vi "Send Publisher Instance Return.vi"(8 "error in (no error)":errorcluster, 10 "Publisher Instance":T1, 11 "CIFChannelMng in":refnum<class "CIFChannelMng.lvclass">) -> (0 "error out":errorcluster, 3 "CIFChannelMng out":refnum<class "CIFChannelMng.lvclass">)   [LabVIEW 2021, in "CIFChannelMng.lvclass"]
uses:
  CIFChannelMng.lvclass
  OOB/OOB_Tx/Typedef/FIFO Publisher Return.ctl
  CIFChannelMng.lvclass/CIFChannelMng.ctl
  <vilib>/CIF Foundation/CIF Out of Band Commands/CIFOutOfBand.lvclass/CIFOutOfBand.ctl
  <vilib>/CIF Foundation/CIF Out of Band Commands/Queue Command.vi
  <vilib>/CIF Foundation/CIF Out of Band Commands/Utilities/Command to Bitwise Command.vi
  <vilib>/CIF Foundation/CIF Out of Band Commands/Accessors/Read Local OOB Data.vi
  OOB/OOB_Tx/ChnMngOOB_Tx.lvclass
  C:/Program Files/National Instruments/LabVIEW 2021/vi.lib/CIF Foundation/CIF Out of Band Commands/CIFOutOfBand.lvclass
  <vilib>/CIF Foundation/CIF Out of Band Commands/CIFOutOfBand.lvclass
  D:/dev/CIF-LVCore/src/Channels/CIFChannelMng/OOB/OOB_Tx/ChnMngOOB_Tx.lvclass
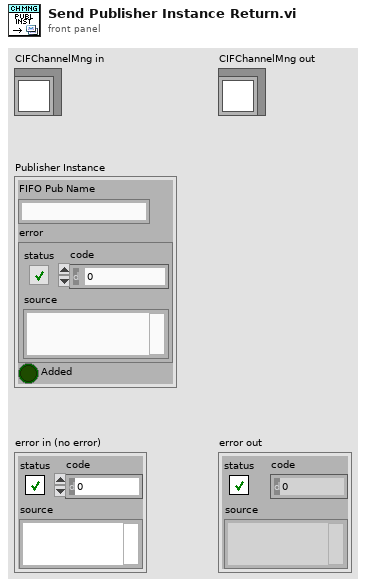
[diagram p1: front panel]
types:
  T1 = typedef "ChnMngOOB_Tx.lvclass/FIFO Publisher Return.ctl" = cluster{"FIFO Pub Name":string, "error":errorcluster, "Added":bool}
  T2 = typedef "CIFChannelMng.lvclass/Channel List for OOB.ctl" = cluster{"Name":string, "Direction":T3, "Type":string, "Connected?":bool, "Connected Name":string, "Custom Config Data":u8[], "Forced?":bool, "Multi-Writer":bool}
  T3 = typedef "CIFChannels.lvclass/Direction.ctl" = enum16{"Publisher", "Subscriber"}
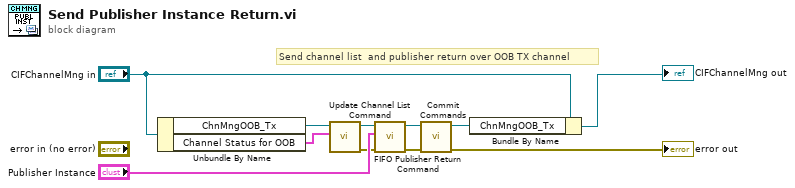
[diagram p0: block diagram]
diagram:
  # "Send channel list  and publisher return over OOB TX channel"
  n1 = Unbundle By Name("CIFChannelMng in") -> ("ChnMngOOB_Tx"=w5:refnum<class "ChnMngOOB_Tx.lvclass">, "Channel Status for OOB"=w4:T2[])
  n2 = call "Update Channel List Command.vi"("Channel List"=w4, "ChanMngOOB_Tx in"=w5) -> ("error out"=w2:errorcluster, "ChanMngOOB_Tx out"=w3:refnum<class "ChnMngOOB_Tx.lvclass">)  [unwired: 8 in]
  n3 = call "FIFO Publisher Return Command.vi"("error in"=w2, "FIFO Publisher"="Publisher Instance", "ChanMngOOB_Tx in"=w3) -> ("error out"=w7:errorcluster, "ChanMngOOB_Tx out"=w8:refnum<class "ChnMngOOB_Tx.lvclass">)  [unwired: 7 in]
  n4 = call <vilib>:"Commit Commands.vi"("error in"=w7, "OOB in"=w8) -> ("error out"=→"error out":errorcluster, "OOB out"=w9:refnum<class "ChnMngOOB_Tx.lvclass">)  [unwired: 8 in]
  n5 = Bundle By Name(cluster="CIFChannelMng in", "ChnMngOOB_Tx"=w9) -> (→"CIFChannelMng out":refnum<class "CIFChannelMng.lvclass">)
